vi "_029.vi"() -> ()   [LabVIEW 2024]
panel:
  in  "stop":bool
  in  "Visible":bool
  in  "Boolean":bool
  # "Property Node :"
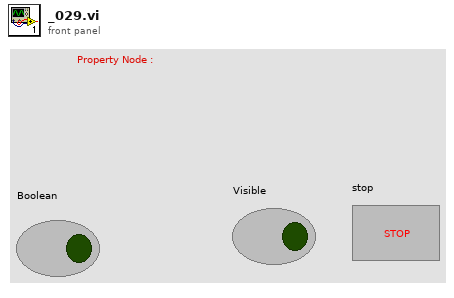
[diagram p1: front panel]
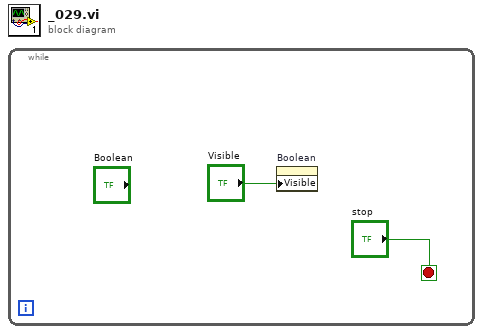
[diagram p0: block diagram]
diagram:
  n1 = while {
    stop <- "stop" stop-if-true
    n2 = property on="Boolean" class="Bool (strict)"("Visible"="Visible") -> ()  [unwired: 2 in, 2 out]
  }
